vi "usernamePassword.vi"() -> ()   [LabVIEW 2021]
uses:
  <vilib>/Utility/file.llb/Read Delimited Spreadsheet (string).vi
panel:
  out "Login Window":string
  in  "Password":string
  in  "Username":string
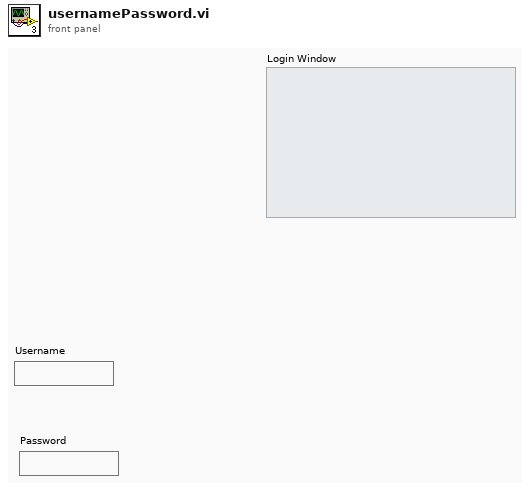
[diagram p1: front panel]
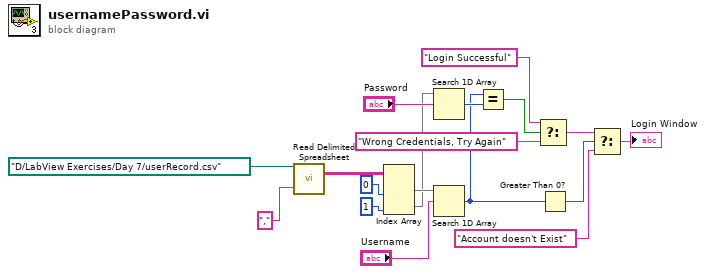
[diagram p0: block diagram]
diagram:
  n1 = call-poly <vilib>:"Read Delimited Spreadsheet.vi"("file path (dialog if empty)"=path "D:/LabView Exercises/Day 7/userRecord.csv" ("File Path"), "delimiter (\\t)"="," ("delimiter (\\t)")) -> ("all rows"=w16:string[][])  [unwired: 8 in, 5 out]
  n2 = Index Array(array=w16, index (col) #1=0 ("disabled index (col)"), index (col) #2=1 ("index (col)")) -> (element #1=w11:string[], element #2=w10:string[])  [unwired: 2 in]
  n3 = Search 1D Array(1D array=w10, element="Password") -> (index of element=w9:i32)  [unwired: 1 in]
  n4 = Search 1D Array(1D array=w11, element="Username") -> (index of element=w8:i32)  [unwired: 1 in]
  n5 = Equal?(x=w8, y=w9) -> (x = y?=w6:bool)
  n6 = Select(t="Login Successful", s=w6, f="Wrong Credentials, Try Again") -> (s? t:f=w2:string)
  n7 = Greater Than 0?(x=w8) -> (x > 0?=w7:bool)
  n8 = Select(t=w2, s=w7, f="Account doesn't Exist" ("t")) -> (s? t:f=→"Login Window":string)
